vi "Set_Disabled.vi"(8 "error in (no error)":errorcluster, 9 "State (0=enabled)":u8=1, 10 "Control Label":string, 11 "CtlLookup In":T1) -> (0 "error out":errorcluster, 3 "CtlLookup Out":T1)   [LabVIEW 2020, in "CtlReferences.lvlib" / "CtlReferences.lvclass"]
doc: "Set disabled state of specified control\n0 = Enabled\n1 = Disabled\n2 = Disabled & Greyed Out"
uses:
  CtlReferences.lvclass
  CtlReferences.lvclass/CtlReferences.ctl
  GetControlRef/GetControl_Control.vi
  TypeDefs/CtlLookup.ctl
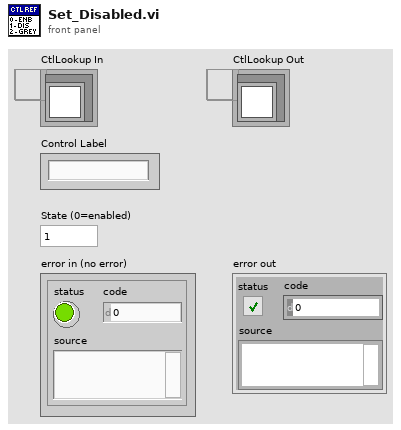
[diagram p1: front panel]
types:
  T1 = typedef "CtlReferences.lvlib/CtlReferences.lvclass/CtlLookup.ctl" = refnum<data-value>
  T2 = enum8{"Enabled", "Disabled", "Disabled and Grayed Out"}
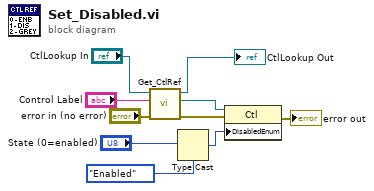
[diagram p0: block diagram]
diagram:
  n1 = call-poly "Get_CtlRef.vi"("error in (no error)"="error in (no error)", "Control Label"="Control Label", "CtlLookup In"="CtlLookup In") -> ("error out"=w8:errorcluster, "Reference Out"=w7:refnum<vi>, "CtlLookup Out"=→"CtlLookup Out":T1)  [unwired: 6 in]
  n2 = Type Cast(type=T2."Enabled" ("Disabled"), x="State (0=enabled)") -> (*(type *) &x=w5:T2)
  n3 = property class="Ctl"(reference=w7, error in=w8, "DisabledEnum"=w5) -> (error out=→"error out":errorcluster)  [unwired: 1 out]
